vi "TestTileAutomation.vi"() -> ()   [LabVIEW 2016]
uses:
  TTA_Controls/TTA_Control_RFIC_List.ctl
  TTA_Controls/TTA_Control_Complete_Settings_Cluster.ctl
  TTA_Globals/Test_Environment.vi
  TTA_Globals/TTA_Instrument_Cluster.vi
  TTA_Globals/TTA_Global_Working_Directory.vi
  TTA_Globals/Test_Status.vi
  TTA_Globals/TTA_Global_Complete_Settings.vi
panel:
  out "MXG VISA":refnum<visa-resource-name>
  out "EXA VISA":refnum<visa-resource-name>
  out "Complete Settings Cluster":T1
  out "Test Status":string
  out "Working Directory":path
  out "error out":errorcluster
  in  "error in (no error)":errorcluster
  in  "Run System":bool
  in  "stop":bool
  in  "Clear All":bool
  in  "TTA Tab Control":T2(tab)
  in  "Test ALL":bool
  in  "RFIC\nChannel Cluster":cluster{"Channel 1":bool, "Channel 2":bool}
  in  "RFIC List":T3
  in  "Test RFIC":bool
  in  "Keep RF Cal":bool
  in  "Load Settings":bool
  in  "Instruments/Criteria Settings File":path
  in  "Generate Report":bool
  in  "Report Path":path
  in  "Test Rx":bool
  in  "Rx\nChannel Cluster":cluster{"Channel 1":bool, "Channel 2":bool}
  in  "Rx List":T3 caption="RFIC List"
  in  "Test Tx":bool
  in  "Tx\nChannel Cluster":cluster{"Channel 1":bool, "Channel 2":bool}
  in  "Tx List":T3 caption="RFIC List"
  in  "TTA COM Port":refnum<visa-resource-name>
  in  "EXA IP Address":string
  in  "MXG IP Address":string
  in  "Serial Number":string caption="Device Under Test"
  in  "MATLAB Path":path=path "C:/Users/Alex.Minicozzi.NJ01/Documents/LabVIEW Data/BDS_MATLAB/ViennaGUI"
  in  "MXG Test \nConnection":bool
  in  "EXA Test \nConnection":bool
  in  "Run Calibration Routine":bool
  out "TxOffset Cal Cluster":T4
  out "RxOffset Cal Cluster":T5
  out "Tx Output Power Criteria Cluster":T6
  out "Rx Output Power Criteria Cluster":T7
  out "TX Output Power Settings Cluster":T8
  out "PAL Calibration\nInputs Cluster":T9
  out "Rx Received Power Settings Cluster":T10
  out "Power Cal Cluster":T11
  out "Tx ACPR Settings Cluster":T12
  out "Brief Cluster":T13
  out "Instrument Setting Cluster":T14
  # "RFIC"
  # "Tx"
  # "Test Description"
  # "Enable"
  # "Channel 1"
  # "Channel 2"
  # "Test Description"
  # "Enable"
  # "Channel 1"
  # "Channel 2"
  # "Rx"
  # "Test Description"
  # "Enable"
  # "Channel 1"
  # "Channel 2"
  # "Tx ACPR"
  # "Tx"
  # "Rx"
  # "Power-Cal"
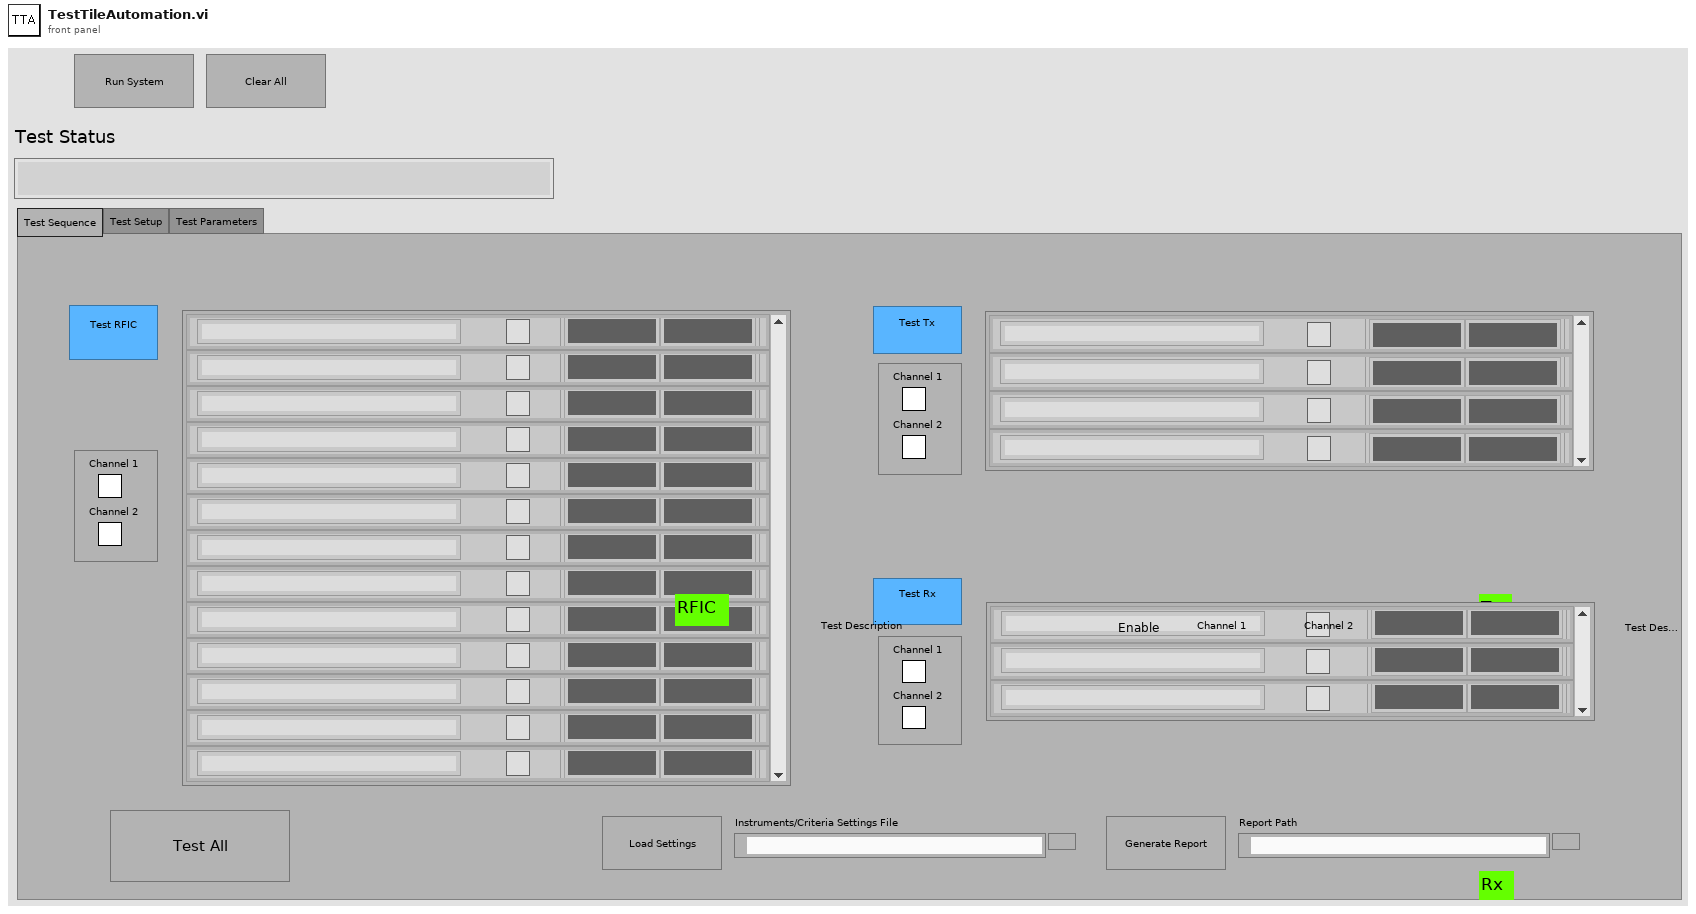
[diagram p1: front panel]
types:
  T1 = typedef "TTA_Control_Complete_Settings_Cluster.ctl" = cluster{"Brief Cluster":cluster{"STM Firmware File":string, "STM Firmware Address":string, "Required SW Version":string, "Template Used":string}, "Instrument Setting Cluster":cluster{"BDSFreq":dbl, "BDS Amp":dbl, "TxRFCal_Freq":dbl, "TxRFCal_Amp":dbl, "RxRFCal_Freq":dbl, "RxRFCal_Freq":dbl, "TxIF_Freq":dbl, "TxIF_Amp":dbl, "Tx_Output_Power_Signal_Freq":dbl, "Tx_ACPR_Signal_Freq":dbl, "Rx_RF_Freq":dbl, "Rx_RF_Amp":dbl, "Rx_Output_Power_Signal_Freq":dbl, "Rx_Output_Power_Sense_Freq":dbl}, "PAL Calibration\nInputs Cluster":cluster{"Amplitude Range\nMax(dBm)":dbl, "Amplitude Range\nMin(dBm)":dbl, "Amplitude Least\nCriteria (dBm)":dbl, "Frequency 1":dbl, "Frequency 2":dbl, "Frequency 3":dbl, "CAL Amplitude\nDecrement (dB)":dbl, "CAL Amplitude\nIncrement(dB)":dbl, "DownloadFile":string}, "TxOffset Cal Cluster":cluster{"Tx1 Offset (dB)":dbl, "Tx2 Offset (dB)":dbl, "Tx3 Offset (dB)":dbl, "Tx4 Offset (dB)":dbl, "Total RF Tx Loss (dB)":dbl}, "RxOffset Cal Cluster":cluster{"Rx1 Offset (dB)":dbl, "Rx2 Offset (dB)":dbl, "Rx3 Offset (dB)":dbl, "Rx4 Offset (dB)":dbl, "Total RF Rx Loss (dB)":dbl}, "TX Output Power Settings Cluster":cluster{"Frequency Sweep (MHz)":dbl[], "Sig Gen \nPower (dBm)":dbl, "Span (kHz)":dbl, "RBW (Hz)":dbl, "Ref Level (dBm)":dbl, "Low Power \nLimit":dbl, "High Power \nLimit":dbl, "DigAtt Max":dbl, "DigAtt Min":dbl}, "Tx ACPR Settings Cluster":cluster{"ACPR Filename":string, "Sampling Rate":dbl, "Power (dBm)":dbl, "IF Frequency Sweep (MHz)":dbl[], "State Name":string, "Mechanical\nAttenuation":dbl, "RefLevel Offset":dbl, "Amplitude Range\nMax (dBm)":dbl, "Amplitude Range\nMin (dBm)":dbl, "Cal Amp \nIncrement (dB)":dbl, "Cal Amp\nDecrement (dB)":dbl}, "Power Cal Cluster":cluster{"Power List (dBm)":dbl[], "Frequency (MHz)":dbl[], "Cal Decrement (dB)":dbl, "Cal Increment (dB)":dbl}, "Rx Received Power Settings Cluster":cluster{"Frequency Sweep (MHz)":dbl[], "Power (dBm)":dbl, "Span (kHz)":dbl, "RBW (Hz)":dbl, "Ref Level":dbl, "Low Power \nLimit (dBm)":dbl, "High Power\nLimit (dBm)":dbl}, "Tx Output Power Criteria Cluster":cluster{"CH1-TX1 \nMin":dbl, "CH1-TX1\nMax":dbl, "CH1-TXx3\nMin ":dbl, "CH1-TXx3\nMax":dbl, "CH2-TX1\nMin":dbl, "CH2-TX1\nMax":dbl, "CH2-TXx3\nMin":dbl, "CH2-TXx3\nMax":dbl}, "Tx ACPR Criteria Cluster":cluster{"Min Inband":dbl, "Max Close Outband":dbl, "Max Far Outband":dbl}, "Rx Output Power Criteria Cluster":cluster{"CH1-RX1 \nMin":dbl, "CH1-RX1 \nMax":dbl, "CH1-RXx3 \nMin":dbl, "CH1-RXx3\nMax":dbl, "CH2-RX1\nMin":dbl, "CH2-RX1\nMax":dbl, "CH2-RXx3\nMin":dbl, "CH2-RXx3\nMax":dbl}}
  T2 = enum32{"Test Sequence", "Test Setup", "Test Parameters"}
  T3 = typedef "TTA_Control_RFIC_List.ctl" = cluster{"Enable":bool, "Test Description":string, "Status Array":u16[]}[]
  T4 = cluster{"Tx1 Offset (dB)":dbl, "Tx2 Offset (dB)":dbl, "Tx3 Offset (dB)":dbl, "Tx4 Offset (dB)":dbl, "Total RF Tx Loss (dB)":dbl}
  T5 = cluster{"Rx1 Offset (dB)":dbl, "Rx2 Offset (dB)":dbl, "Rx3 Offset (dB)":dbl, "Rx4 Offset (dB)":dbl, "Total RF Rx Loss (dB)":dbl}
  T6 = cluster{"CH1-TX1 \nMin":dbl, "CH1-TX1\nMax":dbl, "CH1-TXx3\nMin ":dbl, "CH1-TXx3\nMax":dbl, "CH2-TX1\nMin":dbl, "CH2-TX1\nMax":dbl, "CH2-TXx3\nMin":dbl, "CH2-TXx3\nMax":dbl}
  T7 = cluster{"CH1-RX1 \nMin":dbl, "CH1-RX1 \nMax":dbl, "CH1-RXx3 \nMin":dbl, "CH1-RXx3\nMax":dbl, "CH2-RX1\nMin":dbl, "CH2-RX1\nMax":dbl, "CH2-RXx3\nMin":dbl, "CH2-RXx3\nMax":dbl}
  T8 = cluster{"Frequency Sweep (MHz)":dbl[], "Sig Gen \nPower (dBm)":dbl, "Span (kHz)":dbl, "RBW (Hz)":dbl, "Ref Level (dBm)":dbl, "Low Power \nLimit":dbl, "High Power \nLimit":dbl, "DigAtt Max":dbl, "DigAtt Min":dbl}
  T9 = cluster{"Amplitude Range\nMax(dBm)":dbl, "Amplitude Range\nMin(dBm)":dbl, "Amplitude Least\nCriteria (dBm)":dbl, "Frequency 1":dbl, "Frequency 2":dbl, "Frequency 3":dbl, "CAL Amplitude\nDecrement (dB)":dbl, "CAL Amplitude\nIncrement(dB)":dbl, "DownloadFile":string}
  T10 = cluster{"Frequency Sweep (MHz)":dbl[], "Power (dBm)":dbl, "Span (kHz)":dbl, "RBW (Hz)":dbl, "Ref Level":dbl, "Low Power \nLimit (dBm)":dbl, "High Power\nLimit (dBm)":dbl}
  T11 = cluster{"Power List (dBm)":dbl[], "Frequency (MHz)":dbl[], "Cal Decrement (dB)":dbl, "Cal Increment (dB)":dbl}
  T12 = cluster{"ACPR Filename":string, "Sampling Rate":dbl, "Power (dBm)":dbl, "IF Frequency Sweep (MHz)":dbl[], "State Name":string, "Mechanical\nAttenuation":dbl, "RefLevel Offset":dbl, "Amplitude Range\nMax (dBm)":dbl, "Amplitude Range\nMin (dBm)":dbl, "Cal Amp \nIncrement (dB)":dbl, "Cal Amp\nDecrement (dB)":dbl}
  T13 = cluster{"STM Firmware File":string, "STM Firmware Address":string, "Required SW Version":string, "Template Used":string}
  T14 = cluster{"BDSFreq":dbl, "BDS Amp":dbl, "TxRFCal_Freq":dbl, "TxRFCal_Amp":dbl, "RxRFCal_Freq":dbl, "RxRFCal_Freq":dbl, "TxIF_Freq":dbl, "TxIF_Amp":dbl, "Tx_Output_Power_Signal_Freq":dbl, "Tx_ACPR_Signal_Freq":dbl, "Rx_RF_Freq":dbl, "Rx_RF_Amp":dbl, "Rx_Output_Power_Signal_Freq":dbl, "Rx_Output_Power_Sense_Freq":dbl}
  T15 = cluster{"VISA resource name":refnum<visa-resource-name>, "VISA resource name":refnum<visa-resource-name>, "TTA COM Port":refnum<visa-resource-name>}
  T16 = cluster{"Enable":bool, "Test Description":string, u16[]}
  T17 = cluster{"EXA VISA Resource":refnum<visa-resource-name>, "MXG VISA Resource":refnum<visa-resource-name>, "TTA COM Port":refnum<visa-resource-name>}
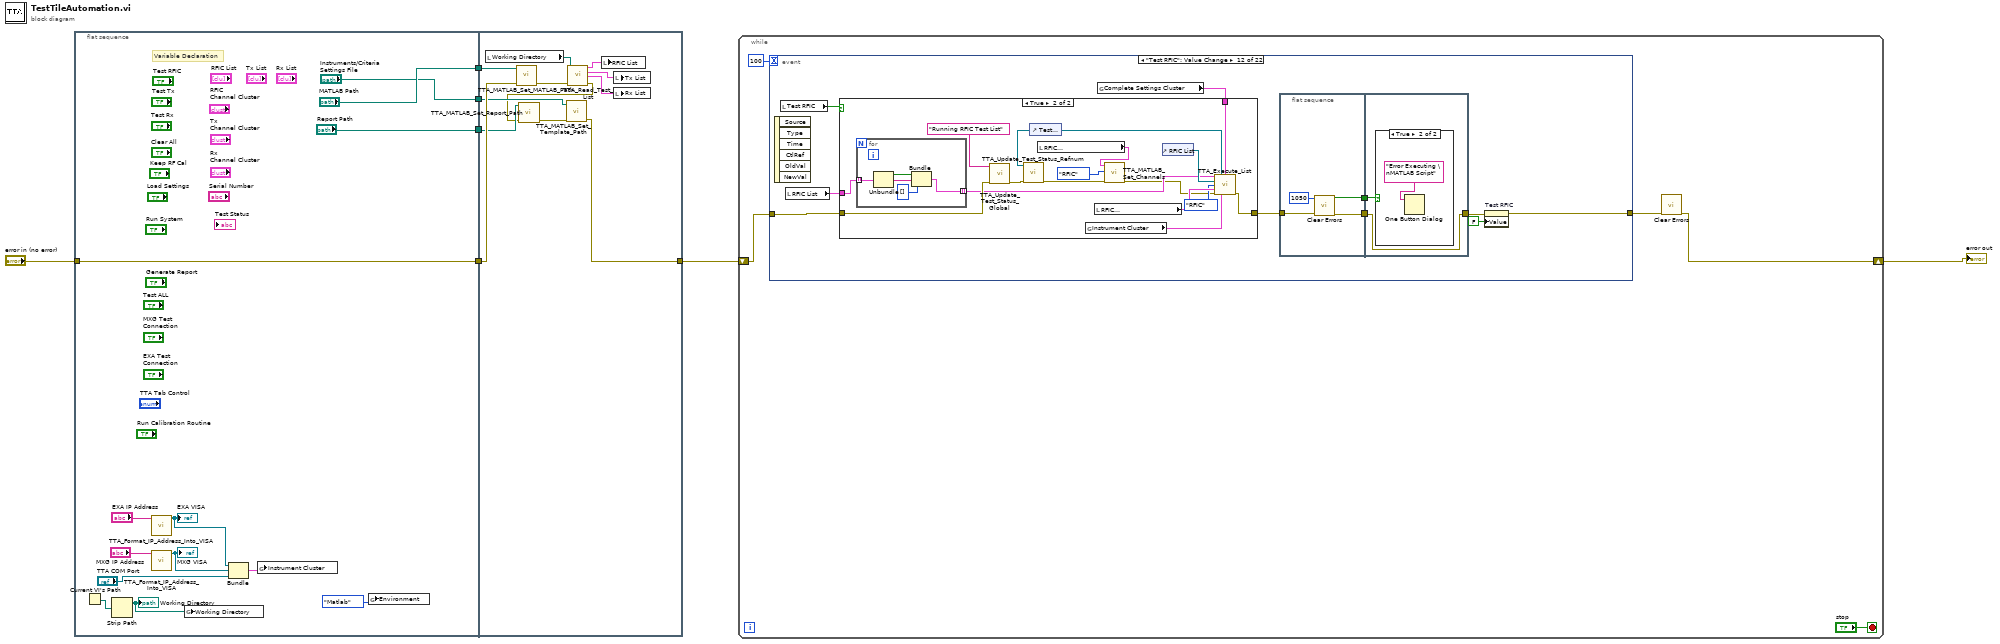
[diagram p0: block diagram]
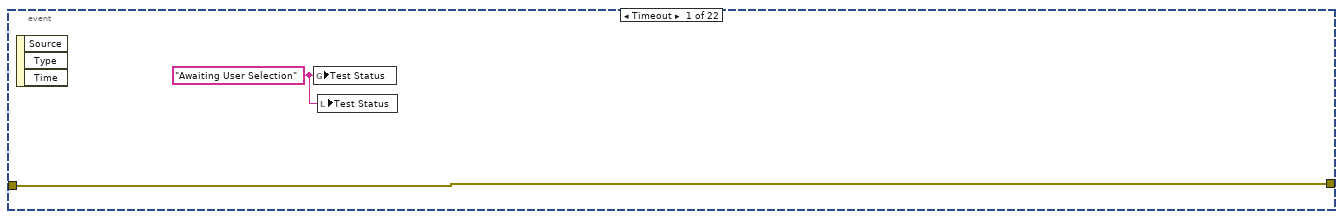
[diagram p2: hidden frame]
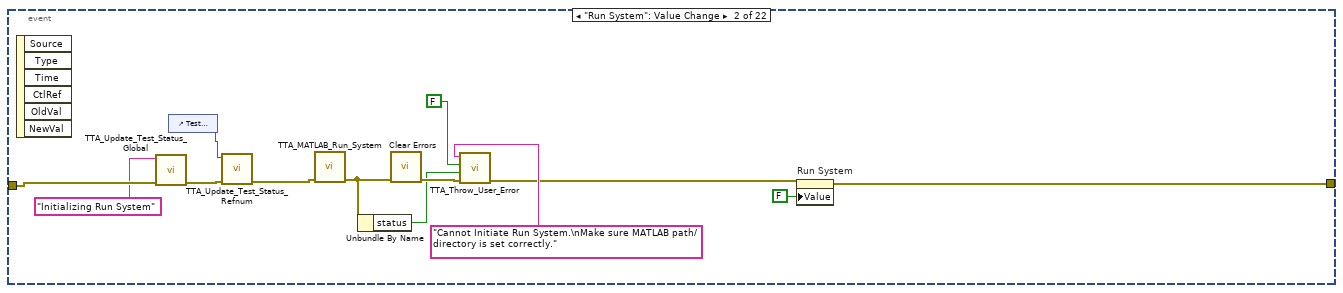
[diagram p3: hidden frame]
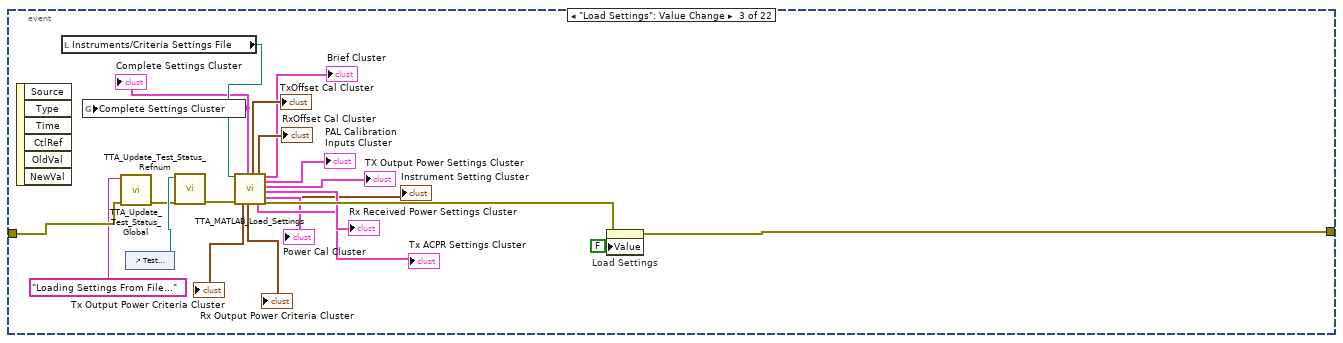
[diagram p4: hidden frame]
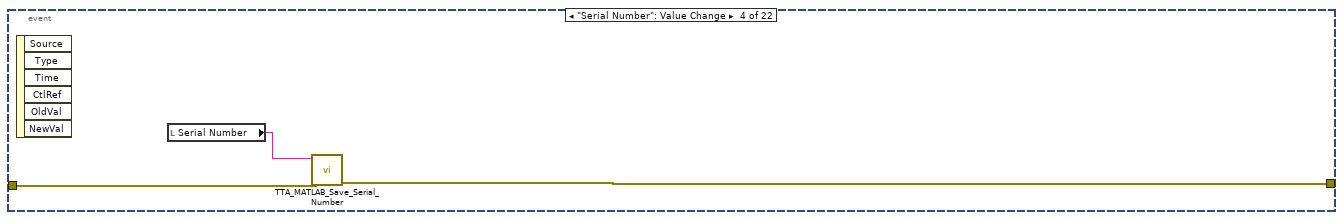
[diagram p5: hidden frame]
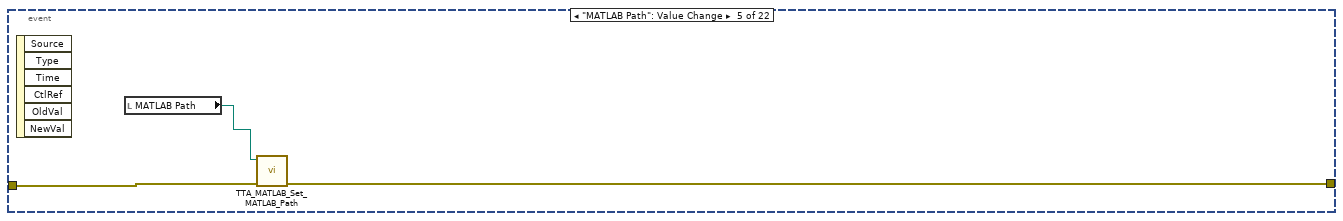
[diagram p6: hidden frame]
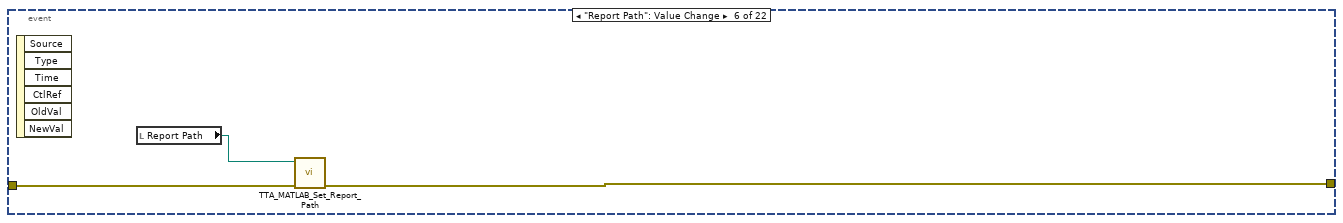
[diagram p7: hidden frame]
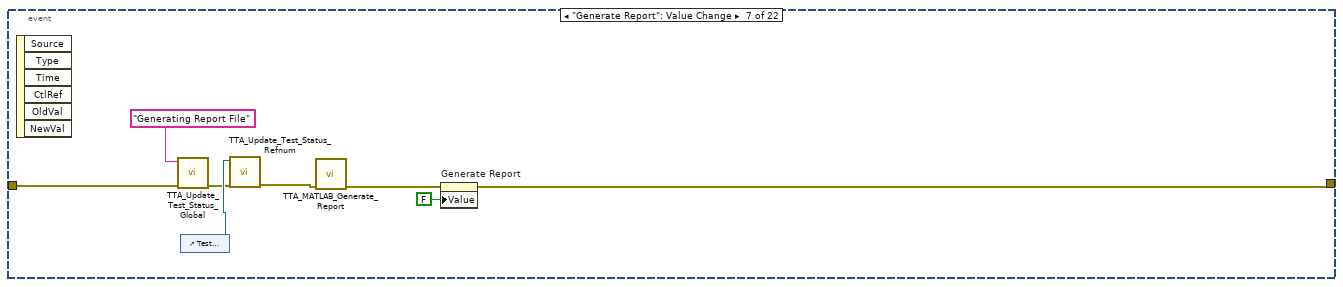
[diagram p8: hidden frame]
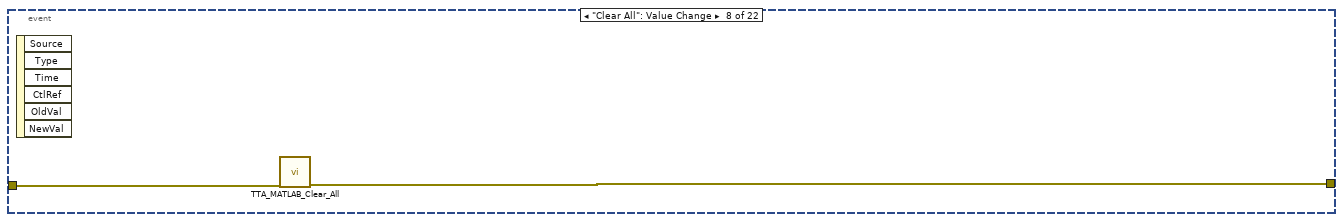
[diagram p9: hidden frame]
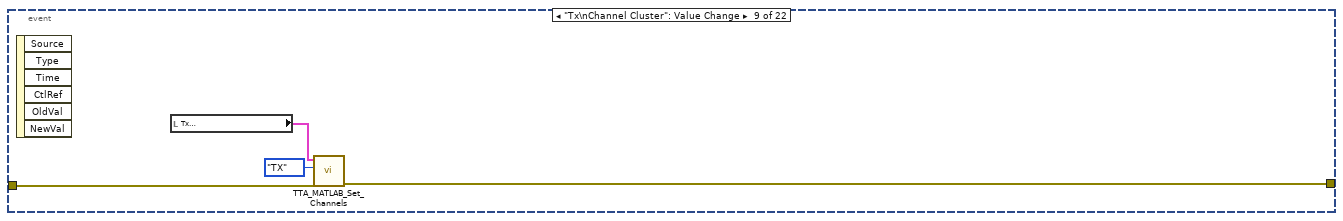
[diagram p10: hidden frame]
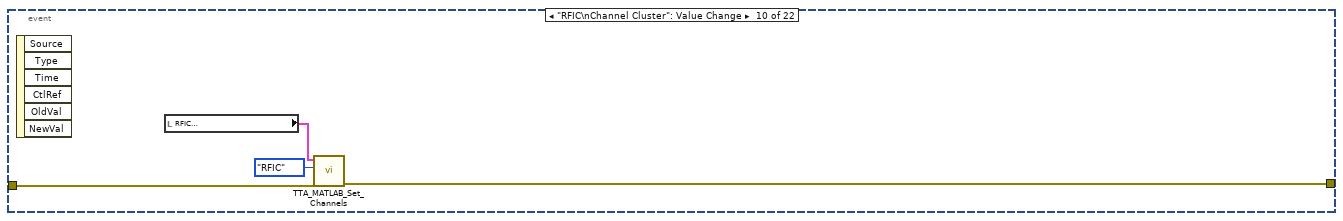
[diagram p11: hidden frame]
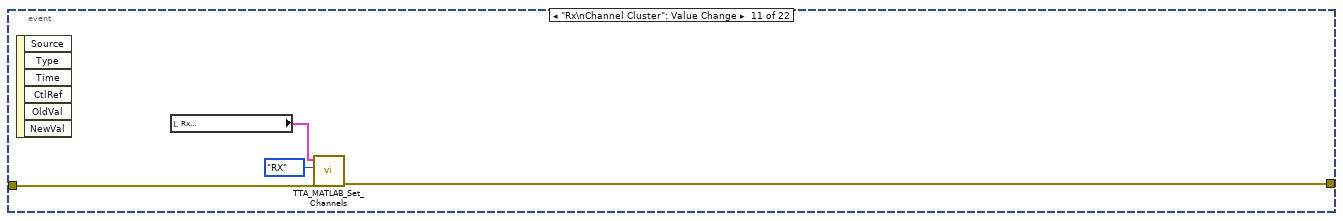
[diagram p12: hidden frame]
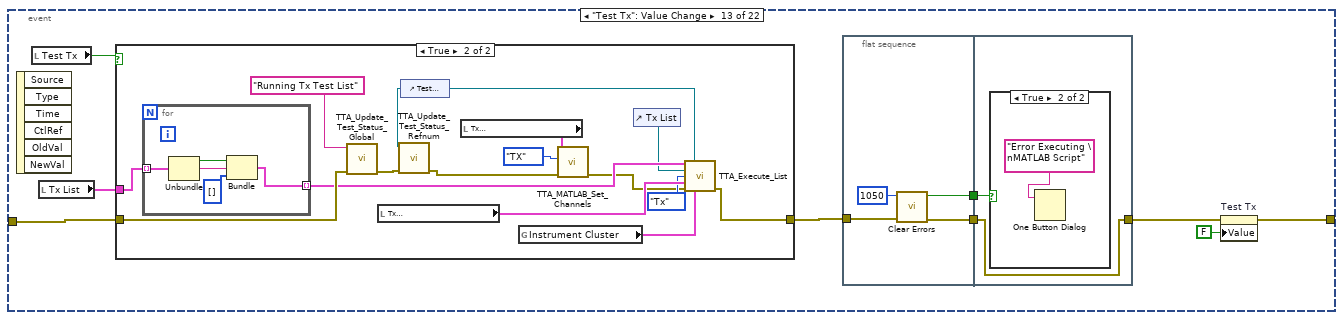
[diagram p15: hidden frame]
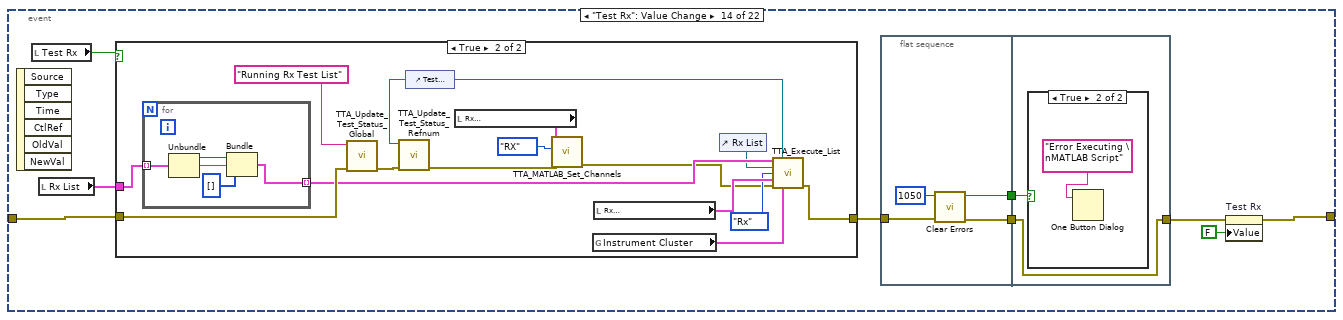
[diagram p18: hidden frame]
diagram:
  n1 = flat-sequence {
    tunnel: "error in (no error)" -> [w20]
    tunnel: [w20] -> w4
    tunnel: ["MATLAB Path"] -> w3
    tunnel: ["Report Path"] -> w2
    tunnel: ["Instruments/Criteria Settings File"] -> w1
    tunnel: [w21] -> w6
    tunnel: w4 -> [w32]
    tunnel: w3 -> [w26]
    tunnel: w2 -> [w25]
    tunnel: w1 -> [w24]
    frame #0 {
      # "Variable Declaration"
      n2 = Current VI's Path() -> (path=w19:path)
      n3 = Strip Path(path=w19) -> (stripped path=w8:path)  [unwired: 1 out]
      "Working Directory" <- w8
      n4 = call "TTA_Format_IP_Address_Into_VISA.vi"("IP Address"="EXA IP Address") -> ("VISA resource name"=w12:refnum<visa-resource-name>)  [unwired: 9 in, 1 out]
      "EXA VISA" <- w12
      n5 = call "TTA_Format_IP_Address_Into_VISA.vi"("IP Address"="MXG IP Address") -> ("VISA resource name"=w11:refnum<visa-resource-name>)  [unwired: 9 in, 1 out]
      "MXG VISA" <- w11
      n6 = global write "TTA_Global_Working_Directory.vi" "Working Directory"(w8) -> ()
      n7 = Bundle("VISA resource name"=w12, "VISA resource name"=w11, "TTA COM Port"="TTA COM Port") -> (w10:T15)  [unwired: 1 in]
      n8 = global write "TTA_Instrument_Cluster.vi" "Instrument Cluster"(w10) -> ()
      n9 = global write "Test_Environment.vi" "Environment"(enum16{"Matlab", "LabVIEW"}."Matlab" ("Environment")) -> ()
    }
    frame #1 {
      n10 = local read "Working Directory"() -> (w29:path)
      n11 = call "TTA_MATLAB_Set_MATLAB_Path.vi"("error in"=w32, "MATLAB Directory"=w26) -> ("error out"=w30:errorcluster)  [unwired: 9 in]
      n12 = call "TTA_Read_Test_List.vi"("Working Directory"=w29, "error in (no error)"=w30) -> ("RFIC List"=w31:T3, "Tx List"=w28:T3, "Rx List"=w27:T3, "error out"=w22:errorcluster)  [unwired: 10 in]
      n13 = call "TTA_MATLAB_Set_Report_Path.vi"("error in"=w22, "Report Directory"=w25) -> ("error out"=w23:errorcluster)  [unwired: 9 in]
      n14 = call "TTA_MATLAB_Set_Template_Path.vi"("error in"=w23, "Template Path"=w24) -> ("error out"=w21:errorcluster)  [unwired: 9 in]
      n15 = local write "RFIC List"(w31) -> ()
      n16 = local write "Tx List"(w28) -> ()
      n17 = local write "Rx List"(w27) -> ()
    }
  }
  n18 = while {
    shift-right: [w33] -> w5
    shift-left: w6 -> [w36]
    stop <- "stop" stop-if-true
    n19 = event shown="[11] \"Test RFIC\": Value Change" {
      selector: _ -> [_ _ _ _ _ _ _ _ _ _ _ _ _ _ _ _ _ _ _ _ _ _]
      dyn-events: _ -> [_ _ _ _ _ _ _ _ _ _ _ _ _ _ _ _ _ _ _ _ _ _]
      timeout: 100 -> [_ _ _ _ _ _ _ _ _ _ _ _ _ _ _ _ _ _ _ _ _ _]
      tunnel: w36 -> [w39 w49 w69 w75 w78 w82 w84 w92 w96 w100 w104 w112 w150 w187 w225 w290 w297 w345 w391 w398 w399 w416]
      tunnel: [w39 w51 w73 w74 w77 w80 w89 w91 w95 w99 w103 w111 w149 w181 w222 w288 w296 w342 w389 w396 w399 w410] -> w34
      event Timeout {
        w38 = "Awaiting User Selection" ("Test Status")
        n20 = event-data() -> ()  [unwired: 1 in, 3 out]
        n21 = global write "Test_Status.vi" "Test Status"(w38) -> ()
        n22 = local write "Test Status"(w38) -> ()
      }
      event "Run System": Value Change {
        n23 = event-data() -> ()  [unwired: 1 in, 6 out]
        n24 = call "TTA_Update_Test_Status_Global.vi"("error in"=w49, "Test Status"="Initializing Run System" ("Status")) -> ("error out"=w50:errorcluster)  [unwired: 9 in]
        n25 = control-ref of="Test Status"() -> (w48:refnum<vi>)
        n26 = call "TTA_Update_Test_Status_Refnum.vi"("error in"=w50, "Test Status Refnum"=w48) -> ("error out"=w46:errorcluster)  [unwired: 9 in]
        n27 = call "TTA_MATLAB_Run_System.vi"("error in"=w46) -> ("error out"=w43:errorcluster)  [unwired: 14 in]
        n28 = Unbundle By Name(w43) -> ("status"=w42:bool)
        n29 = call <vilib>:"Clear Errors.vi"("error in (no error)"=w43) -> ("error out"=w44:errorcluster)  [unwired: 5 in, 1 out]
        n30 = call "TTA_Throw_User_Error.vi"("error in"=w44, "Error?"=w42, "Stop Execution on Fail"=FALSE, "Error Message"="Cannot Initiate Run System.\nMake sure MATLAB path/directory is set correctly.") -> ("error out"=w40:errorcluster)  [unwired: 7 in]
        n31 = property on="Run System" class="Bool (strict)"(error in=w40, "Value"=FALSE ("Run System")) -> (error out=w51:errorcluster)  [unwired: 1 in, 1 out]
      }
      event "Load Settings": Value Change {
        n32 = event-data() -> ()  [unwired: 1 in, 6 out]
        n33 = local read "Instruments/Criteria Settings File"() -> (w71:path)
        n34 = call "TTA_Update_Test_Status_Global.vi"("error in"=w69, "Test Status"="Loading Settings From File..." ("Status")) -> ("error out"=w66:errorcluster)  [unwired: 9 in]
        n35 = control-ref of="Test Status"() -> (w67:refnum<vi>)
        n36 = call "TTA_Update_Test_Status_Refnum.vi"("error in"=w66, "Test Status Refnum"=w67) -> ("error out"=w65:errorcluster)  [unwired: 9 in]
        n37 = call "TTA_MATLAB_Load_Settings.vi"("Instruments/Criteria Settings File"=w71, "error in"=w65) -> ("Tx Output Power Criteria Cluster"=→"Tx Output Power Criteria Cluster":T6, "Complete Settings Cluster"=w53:T1, "Rx Output Power Criteria Cluster"=→"Rx Output Power Criteria Cluster":T7, "TxOffset Cal Cluster"=→"TxOffset Cal Cluster":T4, "Power Cal Cluster"=→"Power Cal Cluster":T11, "RxOffset Cal Cluster"=→"RxOffset Cal Cluster":T5, "Tx ACPR Settings Cluster"=→"Tx ACPR Settings Cluster":T12, "Brief Cluster"=→"Brief Cluster":T13, "PAL Calibration\nInputs Cluster"=→"PAL Calibration\nInputs Cluster":T9, "TX Output Power Settings Cluster"=→"TX Output Power Settings Cluster":T8, "Rx Received Power Settings Cluster"=→"Rx Received Power Settings Cluster":T10, "Instrument Setting Cluster"=→"Instrument Setting Cluster":T14, "error out"=w70:errorcluster)  [unwired: 5 in]
        "Complete Settings Cluster" <- w53
        n38 = global write "TTA_Global_Complete_Settings.vi" "Complete Settings Cluster"(w53) -> ()
        n39 = property on="Load Settings" class="Bool (strict)"(error in=w70, "Value"=FALSE ("Load Settings")) -> (error out=w73:errorcluster)  [unwired: 1 in, 1 out]
      }
      event "Serial Number": Value Change {
        n40 = event-data() -> ()  [unwired: 1 in, 6 out]
        n41 = local read "Serial Number"() -> (w76:string)
        n42 = call "TTA_MATLAB_Save_Serial_Number.vi"("error in"=w75, "Serial Number"=w76) -> ("error out"=w74:errorcluster)  [unwired: 9 in]
      }
      event "MATLAB Path": Value Change {
        n43 = event-data() -> ()  [unwired: 1 in, 6 out]
        n44 = local read "MATLAB Path"() -> (w79:path)
        n45 = call "TTA_MATLAB_Set_MATLAB_Path.vi"("error in"=w78, "MATLAB Directory"=w79) -> ("error out"=w77:errorcluster)  [unwired: 9 in]
      }
      event "Report Path": Value Change {
        n46 = event-data() -> ()  [unwired: 1 in, 6 out]
        n47 = local read "Report Path"() -> (w81:path)
        n48 = call "TTA_MATLAB_Set_Report_Path.vi"("error in"=w82, "Report Directory"=w81) -> ("error out"=w80:errorcluster)  [unwired: 9 in]
      }
      event "Generate Report": Value Change {
        n49 = event-data() -> ()  [unwired: 1 in, 6 out]
        n50 = call "TTA_Update_Test_Status_Global.vi"("error in"=w84, "Test Status"="Generating Report File" ("Status")) -> ("error out"=w85:errorcluster)  [unwired: 9 in]
        n51 = control-ref of="Test Status"() -> (w86:refnum<vi>)
        n52 = call "TTA_Update_Test_Status_Refnum.vi"("error in"=w85, "Test Status Refnum"=w86) -> ("error out"=w83:errorcluster)  [unwired: 9 in]
        n53 = call "TTA_MATLAB_Generate_Report.vi"("error in"=w83) -> ("error out"=w90:errorcluster)  [unwired: 10 in]
        n54 = property on="Generate Report" class="Bool (strict)"(error in=w90, "Value"=FALSE ("Generate Report")) -> (error out=w89:errorcluster)  [unwired: 1 in, 1 out]
      }
      event "Clear All": Value Change {
        n55 = event-data() -> ()  [unwired: 1 in, 6 out]
        n56 = call "TTA_MATLAB_Clear_All.vi"("error in"=w92) -> ("error out"=w91:errorcluster)  [unwired: 10 in]
      }
      event "Tx\nChannel Cluster": Value Change {
        n57 = event-data() -> ()  [unwired: 1 in, 6 out]
        n58 = local read "Tx\nChannel Cluster"() -> (w93:cluster{"Channel 1":bool, "Channel 2":bool})
        n59 = call "TTA_MATLAB_Set_Channels.vi"("error in"=w96, "Tile Section"=enum16{"RFIC", "TX", "RX"}."TX", "Channel Cluster"=w93) -> ("error out"=w95:errorcluster)  [unwired: 8 in]
      }
      event "RFIC\nChannel Cluster": Value Change {
        n60 = event-data() -> ()  [unwired: 1 in, 6 out]
        n61 = local read "RFIC\nChannel Cluster"() -> (w97:cluster{"Channel 1":bool, "Channel 2":bool})
        n62 = call "TTA_MATLAB_Set_Channels.vi"("error in"=w100, "Tile Section"=enum16{"RFIC", "TX", "RX"}."RFIC", "Channel Cluster"=w97) -> ("error out"=w99:errorcluster)  [unwired: 8 in]
      }
      event "Rx\nChannel Cluster": Value Change {
        n63 = event-data() -> ()  [unwired: 1 in, 6 out]
        n64 = local read "Rx\nChannel Cluster"() -> (w101:cluster{"Channel 1":bool, "Channel 2":bool})
        n65 = call "TTA_MATLAB_Set_Channels.vi"("error in"=w104, "Tile Section"=enum16{"RFIC", "TX", "RX"}."RX", "Channel Cluster"=w101) -> ("error out"=w103:errorcluster)  [unwired: 8 in]
      }
      event "Test RFIC": Value Change {
        n66 = event-data() -> ()  [unwired: 1 in, 6 out]
        n67 = local read "Test RFIC"() -> (w114:bool)
        n68 = local read "RFIC List"() -> (w113:T3)
        n69 = global read "TTA_Global_Complete_Settings.vi" "Complete Settings Cluster"() -> (w107:T1)
        n70 = case shown="True" w114 {
          tunnel: w113 -> [_ w132]
          tunnel: w112 -> [w122 w134]
          tunnel: [w122 w138] -> w109
          tunnel: w107 -> [_ w124]
          frame False {
          }
          frame True {
            n71 = for {
              tunnel: w132 -> [w143] mode=indexing
              tunnel: [w140] -> w131 mode=indexing
              n72 = Unbundle(w143) -> ("Enable"=w142:bool, "Test Description"=w141:string)  [unwired: 1 out]
              n73 = Bundle("Enable"=w142, "Test Description"=w141, u16[] []) -> (w140:T16)  [unwired: 1 in]
            }
            n74 = call "TTA_Update_Test_Status_Global.vi"("error in"=w134, "Test Status"="Running RFIC Test List" ("Status")) -> ("error out"=w136:errorcluster)  [unwired: 9 in]
            n75 = control-ref of="Test Status"() -> (w125:refnum<vi>)
            n76 = call "TTA_Update_Test_Status_Refnum.vi"("error in"=w136, "Test Status Refnum"=w125) -> ("error out"=w129:errorcluster)  [unwired: 9 in]
            n77 = local read "RFIC\nChannel Cluster"() -> (w127:cluster{"Channel 1":bool, "Channel 2":bool})
            n78 = global read "TTA_Instrument_Cluster.vi" "Instrument Cluster"() -> (w123:T17)
            n79 = local read "RFIC\nChannel Cluster"() -> (w133:cluster{"Channel 1":bool, "Channel 2":bool})
            n80 = call "TTA_MATLAB_Set_Channels.vi"("error in"=w129, "Tile Section"=enum16{"RFIC", "TX", "RX"}."RFIC", "Channel Cluster"=w127) -> ("error out"=w126:errorcluster)  [unwired: 8 in]
            n81 = control-ref of="RFIC List"() -> (w137:refnum<vi>)
            n82 = call "TTA_Execute_List.vi"("Section List"=w131, "Test Status Refnum"=w125, "Complete Settings Cluster"=w124, "TTA FP\nRFIC Refnum In"=w137, "Tile Section"=enum16{"RFIC", "Tx", "Rx"}."RFIC", "Channel Cluster"=w133, "error in"=w126, "Instrument Cluster In"=w123) -> ("error out"=w138:errorcluster)  [unwired: 7 in]
          }
        }
        n83 = flat-sequence {
          tunnel: w109 -> [w118]
          tunnel: [w117] -> w106
          tunnel: [w115] -> w105
          tunnel: [w119] -> w108
          tunnel: w106 -> [w119]
          tunnel: w105 -> [w120]
          frame #0 {
            n84 = call <vilib>:"Clear Errors.vi"("error in (no error)"=w118, "specific error code to clear (0: all)"=1050) -> ("error out"=w117:errorcluster, "specific error cleared?"=w115:bool)  [unwired: 4 in]
          }
          frame #1 {
            n85 = case shown="True" w120 {
              frame False {
              }
              frame True {
                n86 = One Button Dialog(message="Error Executing \nMATLAB Script") -> ()  [unwired: 1 in, 1 out]
              }
            }
          }
        }
        n87 = property on="Test RFIC" class="Bool (strict)"(error in=w108, "Value"=FALSE ("Test RFIC")) -> (error out=w111:errorcluster)  [unwired: 1 in, 1 out]
      }
      event "Test Tx": Value Change {
        n88 = event-data() -> ()  [unwired: 1 in, 6 out]
        n89 = local read "Test Tx"() -> (w152:bool)
        n90 = local read "Tx List"() -> (w151:T3)
        n91 = case shown="True" w152 {
          tunnel: w151 -> [_ w170]
          tunnel: w150 -> [w160 w172]
          tunnel: [w160 w175] -> w145
          frame False {
          }
          frame True {
            n92 = for {
              tunnel: w170 -> [w180] mode=indexing
              tunnel: [w177] -> w169 mode=indexing
              n93 = Unbundle(w180) -> ("Enable"=w179:bool, "Test Description"=w178:string)  [unwired: 1 out]
              n94 = Bundle("Enable"=w179, "Test Description"=w178, u16[] []) -> (w177:T16)  [unwired: 1 in]
            }
            n95 = call "TTA_Update_Test_Status_Global.vi"("error in"=w172, "Test Status"="Running Tx Test List" ("Status")) -> ("error out"=w174:errorcluster)  [unwired: 9 in]
            n96 = local read "Tx\nChannel Cluster"() -> (w171:cluster{"Channel 1":bool, "Channel 2":bool})
            n97 = control-ref of="Test Status"() -> (w166:refnum<vi>)
            n98 = call "TTA_Update_Test_Status_Refnum.vi"("error in"=w174, "Test Status Refnum"=w166) -> ("error out"=w163:errorcluster)  [unwired: 9 in]
            n99 = local read "Tx\nChannel Cluster"() -> (w164:cluster{"Channel 1":bool, "Channel 2":bool})
            n100 = global read "TTA_Instrument_Cluster.vi" "Instrument Cluster"() -> (w161:T17)
            n101 = call "TTA_MATLAB_Set_Channels.vi"("error in"=w163, "Tile Section"=enum16{"RFIC", "TX", "RX"}."TX", "Channel Cluster"=w164) -> ("error out"=w162:errorcluster)  [unwired: 8 in]
            n102 = control-ref of="Tx List"() -> (w168:refnum<vi>)
            n103 = call "TTA_Execute_List.vi"("Section List"=w169, "Test Status Refnum"=w166, "TTA FP\nRFIC Refnum In"=w168, "Tile Section"=enum16{"RFIC", "Tx", "Rx"}."Tx", "Channel Cluster"=w171, "error in"=w162, "Instrument Cluster In"=w161) -> ("error out"=w175:errorcluster)  [unwired: 8 in]
          }
        }
        n104 = flat-sequence {
          tunnel: w145 -> [w156]
          tunnel: [w155] -> w147
          tunnel: [w153] -> w146
          tunnel: [w157] -> w144
          tunnel: w147 -> [w157]
          tunnel: w146 -> [w158]
          frame #0 {
            n105 = call <vilib>:"Clear Errors.vi"("error in (no error)"=w156, "specific error code to clear (0: all)"=1050) -> ("error out"=w155:errorcluster, "specific error cleared?"=w153:bool)  [unwired: 4 in]
          }
          frame #1 {
            n106 = case shown="True" w158 {
              frame False {
              }
              frame True {
                n107 = One Button Dialog(message="Error Executing \nMATLAB Script") -> ()  [unwired: 1 in, 1 out]
              }
            }
          }
        }
        n108 = property on="Test Tx" class="Bool (strict)"(error in=w144, "Value"=FALSE ("Test Tx")) -> (error out=w149:errorcluster)  [unwired: 1 in, 1 out]
      }
      event "Test Rx": Value Change {
        n109 = event-data() -> ()  [unwired: 1 in, 6 out]
        n110 = local read "Test Rx"() -> (w189:bool)
        n111 = local read "Rx List"() -> (w188:T3)
        n112 = case shown="True" w189 {
          tunnel: w188 -> [_ w207]
          tunnel: w187 -> [w197 w209]
          tunnel: [w197 w212] -> w184
          frame False {
          }
          frame True {
            n113 = for {
              tunnel: w207 -> [w217] mode=indexing
              tunnel: [w214] -> w206 mode=indexing
              n114 = Unbundle(w217) -> ("Enable"=w216:bool, "Test Description"=w215:string)  [unwired: 1 out]
              n115 = Bundle("Enable"=w216, "Test Description"=w215, u16[] []) -> (w214:T16)  [unwired: 1 in]
            }
            n116 = call "TTA_Update_Test_Status_Global.vi"("error in"=w209, "Test Status"="Running Rx Test List" ("Status")) -> ("error out"=w211:errorcluster)  [unwired: 9 in]
            n117 = control-ref of="Test Status"() -> (w203:refnum<vi>)
            n118 = call "TTA_Update_Test_Status_Refnum.vi"("error in"=w211, "Test Status Refnum"=w203) -> ("error out"=w200:errorcluster)  [unwired: 9 in]
            n119 = local read "Rx\nChannel Cluster"() -> (w201:cluster{"Channel 1":bool, "Channel 2":bool})
            n120 = call "TTA_MATLAB_Set_Channels.vi"("error in"=w200, "Tile Section"=enum16{"RFIC", "TX", "RX"}."RX", "Channel Cluster"=w201) -> ("error out"=w199:errorcluster)  [unwired: 8 in]
            n121 = global read "TTA_Instrument_Cluster.vi" "Instrument Cluster"() -> (w198:T17)
            n122 = local read "Rx\nChannel Cluster"() -> (w208:cluster{"Channel 1":bool, "Channel 2":bool})
            n123 = control-ref of="Rx List"() -> (w205:refnum<vi>)
            n124 = call "TTA_Execute_List.vi"("Section List"=w206, "Test Status Refnum"=w203, "TTA FP\nRFIC Refnum In"=w205, "Tile Section"=enum16{"RFIC", "Tx", "Rx"}."Rx", "Channel Cluster"=w208, "error in"=w199, "Instrument Cluster In"=w198) -> ("error out"=w212:errorcluster)  [unwired: 8 in]
          }
        }
        n125 = flat-sequence {
          tunnel: w184 -> [w193]
          tunnel: [w192] -> w186
          tunnel: [w190] -> w185
          tunnel: [w194] -> w182
          tunnel: w186 -> [w194]
          tunnel: w185 -> [w195]
          frame #0 {
            n126 = call <vilib>:"Clear Errors.vi"("error in (no error)"=w193, "specific error code to clear (0: all)"=1050) -> ("error out"=w192:errorcluster, "specific error cleared?"=w190:bool)  [unwired: 4 in]
          }
          frame #1 {
            n127 = case shown="True" w195 {
              frame False {
              }
              frame True {
                n128 = One Button Dialog(message="Error Executing \nMATLAB Script") -> ()  [unwired: 1 in, 1 out]
              }
            }
          }
        }
        n129 = property on="Test Rx" class="Bool (strict)"(error in=w182, "Value"=FALSE ("Test Rx")) -> (error out=w181:errorcluster)  [unwired: 1 in, 1 out]
      }
      event "Test ALL": Value Change {
        n130 = event-data() -> ()  [unwired: 1 in, 6 out]
        n131 = local read "Test ALL"() -> (w224:bool)
        n132 = case shown="True" w224 {
          tunnel: w225 -> [w233 w235]
          tunnel: [w233 w236] -> w219
          frame False {
          }
          frame True {
            w234 = enum16{"RFIC", "TX", "RX"}[] [enum."RFIC", enum."TX", enum."RX"] items=["RFIC", "TX", "RX"]
            n133 = for {
              tunnel: [w239] -> w236
              tunnel: w235 -> [w238]
              tunnel: w234 -> [w237] mode=indexing
              n134 = case shown="\"TX\"" w237 {
                tunnel: [w250 w266 w282] -> w239
                tunnel: w238 -> [w246 w262 w277]
                frame "TX" {
                  n135 = local read "Tx List"() -> (w241:T3)
                  n136 = for {
                    tunnel: w241 -> [w255] mode=indexing
                    tunnel: [w253] -> w243 mode=indexing
                    n137 = Unbundle(w255) -> ("Test Description"=w254:string)  [unwired: 2 out]
                    n138 = Bundle(TRUE, "Test Description"=w254, u16[] []) -> (w253:cluster{bool, "Test Description":string, u16[]})  [unwired: 1 in]
                  }
                  n139 = local write "Tx List"(w243) -> ()
                  n140 = local read "Tx\nChannel Cluster"() -> (w244:cluster{"Channel 1":bool, "Channel 2":bool})
                  n141 = call "TTA_Update_Test_Status_Global.vi"("error in"=w246, "Test Status"="Running Tx Test List" ("Status")) -> ("error out"=w248:errorcluster)  [unwired: 9 in]
                  n142 = control-ref of="Test Status"() -> (w249:refnum<vi>)
                  n143 = call "TTA_Update_Test_Status_Refnum.vi"("error in"=w248, "Test Status Refnum"=w249) -> ("error out"=w245:errorcluster)  [unwired: 9 in]
                  n144 = control-ref of="Tx List"() -> (w242:refnum<vi>)
                  n145 = call "TTA_Execute_List.vi"("Section List"=w243, "TTA FP\nRFIC Refnum In"=w242, "Tile Section"=enum16{"RFIC", "Tx", "Rx"}."Tx", "Channel Cluster"=w244, "error in"=w245) -> ("error out"=w250:errorcluster)  [unwired: 10 in]
                }
                frame "RX" {
                  n146 = local read "Rx List"() -> (w257:T3)
                  n147 = for {
                    tunnel: w257 -> [w271] mode=indexing
                    tunnel: [w269] -> w259 mode=indexing
                    n148 = Unbundle(w271) -> ("Test Description"=w270:string)  [unwired: 2 out]
                    n149 = Bundle(TRUE, "Test Description"=w270, u16[] []) -> (w269:cluster{bool, "Test Description":string, u16[]})  [unwired: 1 in]
                  }
                  n150 = local write "Rx List"(w259) -> ()
                  n151 = local read "Rx\nChannel Cluster"() -> (w260:cluster{"Channel 1":bool, "Channel 2":bool})
                  n152 = call "TTA_Update_Test_Status_Global.vi"("error in"=w262, "Test Status"="Running Rx Test List" ("Status")) -> ("error out"=w264:errorcluster)  [unwired: 9 in]
                  n153 = control-ref of="Test Status"() -> (w265:refnum<vi>)
                  n154 = call "TTA_Update_Test_Status_Refnum.vi"("error in"=w264, "Test Status Refnum"=w265) -> ("error out"=w261:errorcluster)  [unwired: 9 in]
                  n155 = control-ref of="Rx List"() -> (w258:refnum<vi>)
                  n156 = call "TTA_Execute_List.vi"("Section List"=w259, "TTA FP\nRFIC Refnum In"=w258, "Tile Section"=enum16{"RFIC", "Tx", "Rx"}."Rx", "Channel Cluster"=w260, "error in"=w261) -> ("error out"=w266:errorcluster)  [unwired: 10 in]
                }
                frame "RFIC", Default {
                  n157 = local read "RFIC List"() -> (w273:T3)
                  n158 = for {
                    tunnel: w273 -> [w287] mode=indexing
                    tunnel: [w285] -> w274 mode=indexing
                    n159 = Unbundle(w287) -> ("Test Description"=w286:string)  [unwired: 2 out]
                    n160 = Bundle(TRUE, "Test Description"=w286, u16[] []) -> (w285:cluster{bool, "Test Description":string, u16[]})  [unwired: 1 in]
                  }
                  n161 = local write "RFIC List"(w274) -> ()
                  n162 = local read "RFIC\nChannel Cluster"() -> (w275:cluster{"Channel 1":bool, "Channel 2":bool})
                  n163 = call "TTA_Update_Test_Status_Global.vi"("error in"=w277, "Test Status"="Running RFIC Test List" ("Status")) -> ("error out"=w279:errorcluster)  [unwired: 9 in]
                  n164 = control-ref of="Test Status"() -> (w280:refnum<vi>)
                  n165 = call "TTA_Update_Test_Status_Refnum.vi"("error in"=w279, "Test Status Refnum"=w280) -> ("error out"=w276:errorcluster)  [unwired: 9 in]
                  n166 = control-ref of="RFIC List"() -> (w281:refnum<vi>)
                  n167 = call "TTA_Execute_List.vi"("Section List"=w274, "TTA FP\nRFIC Refnum In"=w281, "Tile Section"=enum16{"RFIC", "Tx", "Rx"}."RFIC", "Channel Cluster"=w275, "error in"=w276) -> ("error out"=w282:errorcluster)  [unwired: 10 in]
                }
              }
            }
          }
        }
        n168 = flat-sequence {
          tunnel: w219 -> [w229]
          tunnel: [w228] -> w221
          tunnel: [w226] -> w220
          tunnel: [w230] -> w218
          tunnel: w221 -> [w230]
          tunnel: w220 -> [w231]
          frame #0 {
            n169 = call <vilib>:"Clear Errors.vi"("error in (no error)"=w229, "specific error code to clear (0: all)"=1050) -> ("error out"=w228:errorcluster, "specific error cleared?"=w226:bool)  [unwired: 4 in]
          }
          frame #1 {
            n170 = case shown="True" w231 {
              frame False {
              }
              frame True {
                n171 = One Button Dialog(message="Error Executing \nMATLAB Script") -> ()  [unwired: 1 in, 1 out]
              }
            }
          }
        }
        n172 = property on="Test ALL" class="Bool (strict)"(error in=w218, "Value"=FALSE ("Test ALL")) -> (error out=w222:errorcluster)  [unwired: 1 in, 1 out]
      }
      event "Instruments/Criteria Settings File": Value Change {
        n173 = event-data() -> ()  [unwired: 1 in, 6 out]
        n174 = local read "Instruments/Criteria Settings File"() -> (w289:path)
        n175 = call "TTA_MATLAB_Set_Template_Path.vi"("error in"=w290, "Template Path"=w289) -> ("error out"=w288:errorcluster)  [unwired: 9 in]
      }
      event "MXG Test \nConnection": Value Change {
        n176 = event-data() -> ("NewVal"=w294:bool)  [unwired: 1 in, 5 out]
        n177 = case shown="True" w294 {
          tunnel: w297 -> [w298 w300]
          tunnel: [w298 w308] -> w293
          tunnel: "Testing MXG Connection" -> [_ w301]
          frame False {
          }
          frame True {
            n178 = flat-sequence {
              tunnel: w301 -> [w311]
              tunnel: w300 -> [w310]
              tunnel: [w309] -> w299
              tunnel: [w316] -> w307
              tunnel: [w315] -> w306
              tunnel: w299 -> [w314]
              tunnel: [w321] -> w305
              tunnel: w307 -> [w320]
              tunnel: w306 -> [w319]
              tunnel: [w318] -> w303
              tunnel: w305 -> [w333]
              tunnel: [w322] -> w304
              tunnel: w303 -> [w332]
              tunnel: [w326] -> w302
              tunnel: w304 -> [w335]
              tunnel: [w335] -> w308
              tunnel: w302 -> [w334]
              frame #0 {
                n179 = call "TTA_Update_Test_Status_Global.vi"("error in"=w310, "Test Status"=w311) -> ("error out"=w312:errorcluster)  [unwired: 9 in]
                n180 = control-ref of="Test Status"() -> (w313:refnum<vi>)
                n181 = call "TTA_Update_Test_Status_Refnum.vi"("error in"=w312, "Test Status Refnum"=w313) -> ("error out"=w309:errorcluster)  [unwired: 9 in]
              }
              frame #1 {
                n182 = local read "MXG IP Address"() -> (w317:string)
                n183 = call "TTA_Format_IP_Address_Into_VISA.vi"("error in"=w314, "IP Address"=w317) -> ("error out"=w315:errorcluster, "VISA resource name"=w316:refnum<visa-resource-name>)  [unwired: 8 in]
              }
              frame #2 {
                n184 = local write "MXG VISA"(w320) -> ()
                n185 = VISA Open(error in (no error)=w319, VISA resource name=w320) -> (VISA resource name=w318:refnum<visa-resource-name>, error out=w321:errorcluster)  [unwired: 3 in]
              }
              frame #3 {
                n186 = VISA Write(VISA resource name=w332, write buffer="*IDN?", error in (no error)=w333) -> (VISA resource name out=w329:refnum<visa-resource-name>, error out=w330:errorcluster)  [unwired: 1 out]
                n187 = VISA Read(VISA resource name=w329, byte count=u32 1000, error in (no error)=w330) -> (VISA resource name out=w323:refnum<visa-resource-name>, read buffer=w325:string, error out=w324:errorcluster)  [unwired: 1 out]
                n188 = VISA Close(VISA resource name=w323, error in (no error)=w324) -> (error out=w322:errorcluster)
                n189 = Format Into String(format string="Connection Successful!\n%s", w325) -> (resulting string=w326:string)  [unwired: 2 in, 1 out]
              }
              frame #4 {
                n190 = Unbundle By Name(w335) -> ("status"=w336:bool)
                n191 = Select(t="Failed Connection.  Check settings or connection.", s=w336, f=w334) -> (s? t:f=w338:string)
                n192 = One Button Dialog(message=w338) -> ()  [unwired: 1 in, 1 out]
              }
            }
          }
        }
        n193 = call <vilib>:"Clear Errors.vi"("error in (no error)"=w293) -> ("error out"=w295:errorcluster)  [unwired: 5 in, 1 out]
        n194 = property on="MXG Test \nConnection" class="Bool (strict)"(error in=w295, "Value"=FALSE ("MXG Test \nConnection")) -> (error out=w296:errorcluster)  [unwired: 1 in, 1 out]
      }
      event "EXA Test \nConnection": Value Change {
        n195 = event-data() -> ("NewVal"=w344:bool)  [unwired: 1 in, 5 out]
        n196 = case shown="True" w344 {
          tunnel: w345 -> [w346 w348]
          tunnel: [w346 w356] -> w343
          tunnel: "Testing EXA Connection" -> [_ w349]
          frame False {
          }
          frame True {
            n197 = flat-sequence {
              tunnel: w349 -> [w359]
              tunnel: w348 -> [w358]
              tunnel: [w357] -> w347
              tunnel: [w364] -> w355
              tunnel: [w363] -> w354
              tunnel: w347 -> [w362]
              tunnel: [w369] -> w353
              tunnel: w355 -> [w368]
              tunnel: w354 -> [w367]
              tunnel: [w366] -> w351
              tunnel: w353 -> [w381]
              tunnel: [w370] -> w352
              tunnel: w351 -> [w380]
              tunnel: [w374] -> w350
              tunnel: w352 -> [w383]
              tunnel: [w383] -> w356
              tunnel: w350 -> [w382]
              frame #0 {
                n198 = call "TTA_Update_Test_Status_Global.vi"("error in"=w358, "Test Status"=w359) -> ("error out"=w360:errorcluster)  [unwired: 9 in]
                n199 = control-ref of="Test Status"() -> (w361:refnum<vi>)
                n200 = call "TTA_Update_Test_Status_Refnum.vi"("error in"=w360, "Test Status Refnum"=w361) -> ("error out"=w357:errorcluster)  [unwired: 9 in]
              }
              frame #1 {
                n201 = local read "EXA IP Address"() -> (w365:string)
                n202 = call "TTA_Format_IP_Address_Into_VISA.vi"("error in"=w362, "IP Address"=w365) -> ("error out"=w363:errorcluster, "VISA resource name"=w364:refnum<visa-resource-name>)  [unwired: 8 in]
              }
              frame #2 {
                n203 = local write "EXA VISA"(w368) -> ()
                n204 = VISA Open(error in (no error)=w367, VISA resource name=w368) -> (VISA resource name=w366:refnum<visa-resource-name>, error out=w369:errorcluster)  [unwired: 3 in]
              }
              frame #3 {
                n205 = VISA Write(VISA resource name=w380, write buffer="*IDN?", error in (no error)=w381) -> (VISA resource name out=w377:refnum<visa-resource-name>, error out=w378:errorcluster)  [unwired: 1 out]
                n206 = VISA Read(VISA resource name=w377, byte count=u32 1000, error in (no error)=w378) -> (VISA resource name out=w371:refnum<visa-resource-name>, read buffer=w373:string, error out=w372:errorcluster)  [unwired: 1 out]
                n207 = VISA Close(VISA resource name=w371, error in (no error)=w372) -> (error out=w370:errorcluster)
                n208 = Format Into String(format string="Connection Successful!\n%s", w373) -> (resulting string=w374:string)  [unwired: 2 in, 1 out]
              }
              frame #4 {
                n209 = Unbundle By Name(w383) -> ("status"=w384:bool)
                n210 = Select(t="Failed Connection.  Check settings or connection.", s=w384, f=w382) -> (s? t:f=w386:string)
                n211 = One Button Dialog(message=w386) -> ()  [unwired: 1 in, 1 out]
              }
            }
          }
        }
        n212 = call <vilib>:"Clear Errors.vi"("error in (no error)"=w343) -> ("error out"=w341:errorcluster)  [unwired: 5 in, 1 out]
        n213 = property on="EXA Test \nConnection" class="Bool (strict)"(error in=w341, "Value"=FALSE ("MXG Test \nConnection")) -> (error out=w342:errorcluster)  [unwired: 1 in, 1 out]
      }
      event "MXG IP Address": Value Change {
        n214 = event-data() -> ()  [unwired: 1 in, 6 out]
        n215 = local read "MXG IP Address"() -> (w392:string)
        n216 = call "TTA_Format_IP_Address_Into_VISA.vi"("error in"=w391, "IP Address"=w392) -> ("error out"=w389:errorcluster, "VISA resource name"=w390:refnum<visa-resource-name>)  [unwired: 8 in]
        n217 = global read "TTA_Instrument_Cluster.vi" "Instrument Cluster"() -> (w388:T17)
        n218 = Bundle By Name(cluster=w388, "MXG VISA Resource"=w390) -> (w387:T17)
        n219 = global write "TTA_Instrument_Cluster.vi" "Instrument Cluster"(w387) -> ()
      }
      event "EXA IP Address": Value Change {
        n220 = event-data() -> ()  [unwired: 1 in, 6 out]
        n221 = local read "EXA IP Address"() -> (w393:string)
        n222 = call "TTA_Format_IP_Address_Into_VISA.vi"("error in"=w398, "IP Address"=w393) -> ("error out"=w396:errorcluster, "VISA resource name"=w397:refnum<visa-resource-name>)  [unwired: 8 in]
        n223 = global read "TTA_Instrument_Cluster.vi" "Instrument Cluster"() -> (w395:T17)
        n224 = Bundle By Name(cluster=w395, "EXA VISA Resource"=w397) -> (w394:T17)
        n225 = global write "TTA_Instrument_Cluster.vi" "Instrument Cluster"(w394) -> ()
      }
      event "TTA COM Port": Value Change {
        n226 = event-data() -> ()  [unwired: 1 in, 6 out]
        n227 = local read "TTA COM Port"() -> (w400:refnum<visa-resource-name>)
        n228 = global read "TTA_Instrument_Cluster.vi" "Instrument Cluster"() -> (w402:T17)
        n229 = Bundle By Name(cluster=w402, "TTA COM Port"=w400) -> (w401:T17)
        n230 = global write "TTA_Instrument_Cluster.vi" "Instrument Cluster"(w401) -> ()
      }
      event "Run Calibration Routine": Value Change {
        n231 = event-data() -> ()  [unwired: 1 in, 6 out]
        n232 = local read "Working Directory"() -> (w418:path)
        n233 = Build Path(base path=w418, name or relative path="TTA_Fixture") -> (appended path=w414:path)
        n234 = Build Path(base path=w414, name or relative path="TTA_Calibration_Routine.vi") -> (appended path=w412:path)
        n235 = Open VI Reference(type specifier VI Refnum (for type only)=refnum<vi> refnum, vi path=w412, error in (no error)=w416) -> (vi reference=w422:refnum<vi>, error out=w419:errorcluster)  [unwired: 3 in]
        n236 = invoke class="VI" method="FP.Open"(reference=w422, error in=w419) -> (reference out=w421:refnum<vi>, error out=w420:errorcluster)  [unwired: 3 in, 3 out]
        n237 = invoke class="VI" method="Run VI"(reference=w421, error in=w420, "Wait until done"=TRUE ("Wait Until Done")) -> (reference out=w409:refnum<vi>, error out=w404:errorcluster)  [unwired: 2 in, 3 out]
        n238 = call <vilib>:"Clear Errors.vi"("error in (no error)"=w404, "specific error code to clear (0: all)"=1039) -> ("error out"=w403:errorcluster)  [unwired: 4 in, 1 out]
        n239 = invoke class="VI" method="FP.Close"(reference=w409, error in=w403) -> (reference out=w407:refnum<vi>, error out=w408:errorcluster)  [unwired: 1 in, 1 out]
        n240 = Close Reference(reference=w407, error in (no error)=w408) -> (error out=w411:errorcluster)
        n241 = invoke on="Run Calibration Routine" class="Bool (strict)" method="Reinit To Default"(error in=w411) -> (error out=w410:errorcluster)  [unwired: 2 in, 2 out]
      }
    }
    n242 = call <vilib>:"Clear Errors.vi"("error in (no error)"=w34) -> ("error out"=w33:errorcluster)  [unwired: 5 in, 1 out]
  }
  "error out" <- w5
